vi "FGV_Analyse binary files.vi"(8 "error in (no error)":errorcluster, 9 "Funct data structure":bool, 11 "Get/Set info & refs":T1) -> (0 "Error out":errorcluster, 1 "Cam Binary Videos paths":path[](array[path]), 2 "Cam Binary Videos Refs":refnum<file>[](array[refnum]), 3 "Frame numbers & locations in each video file":T2[](array[typedef]))   [LabVIEW 2017]
uses:
  Typedefs/Number of frames and locations cluster.ctl
  Functional Imaging Viewer/Typedefs/Get-Set-Clear Control.ctl
  Globals/gl_Time series viewer globals.vi
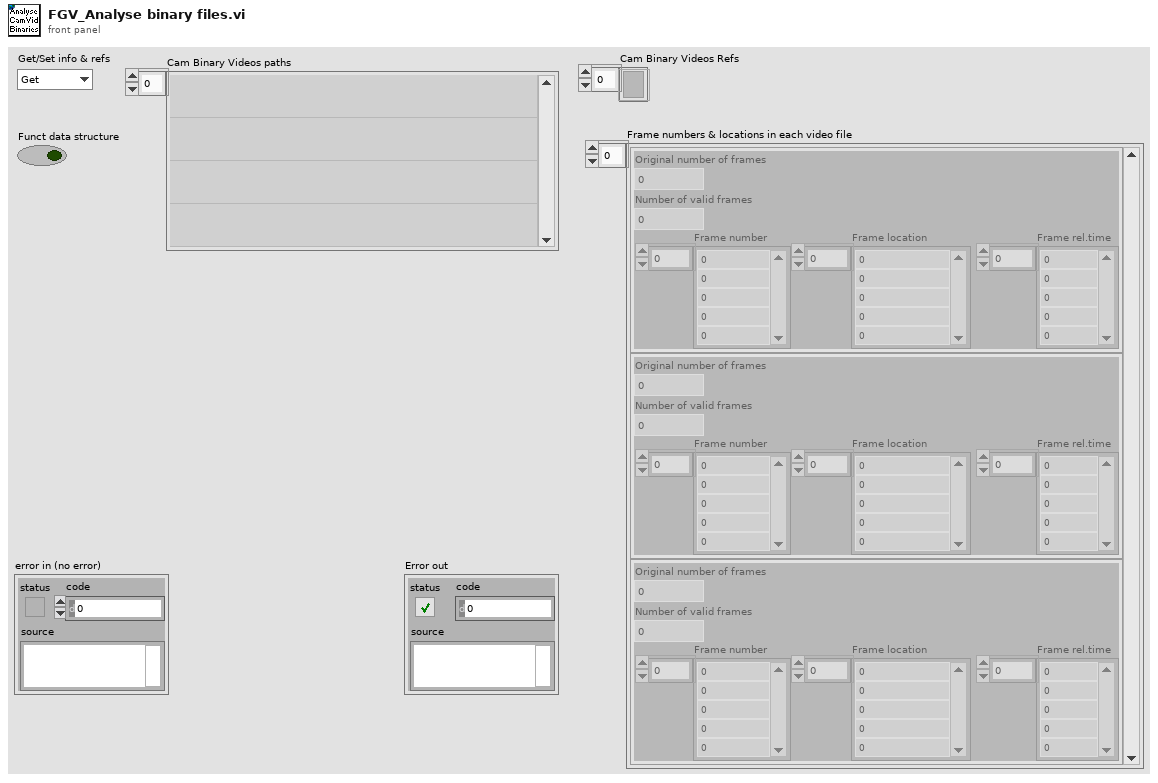
[diagram p1: front panel]
types:
  T1 = typedef "Get-Set-Clear Control.ctl" = enum16{"Get", "Set", "Clear"}
  T2 = typedef "Number of frames and locations cluster.ctl" = cluster{"Original number of frames":i32, "Number of valid frames":i32, "Frame number":i64[], "Frame location":i64[], "Frame rel.time":i64[]}
  T3 = typedef "Time series viewer refs.ctl" = cluster{"This VI":refnum<vi>, "Image control":refnum<vi>, "AVI Mode ind":refnum<vi>, "Play":refnum<vi>, "Stop":refnum<vi>, "Back":refnum<vi>, "Scrollbar":refnum<vi>, "Video length info":refnum<vi>, "Expected speed values":refnum<vi>, "Intensity":refnum<vi>, "Path":refnum<vi>, "Selection sliders":refnum<vi>, "Speed Graph ref":refnum<vi>, "Frame rate set (fps)":refnum<vi>, "Channel to load":refnum<vi>, "Number of rows to generate":refnum<vi>, "Colour":refnum<vi>}
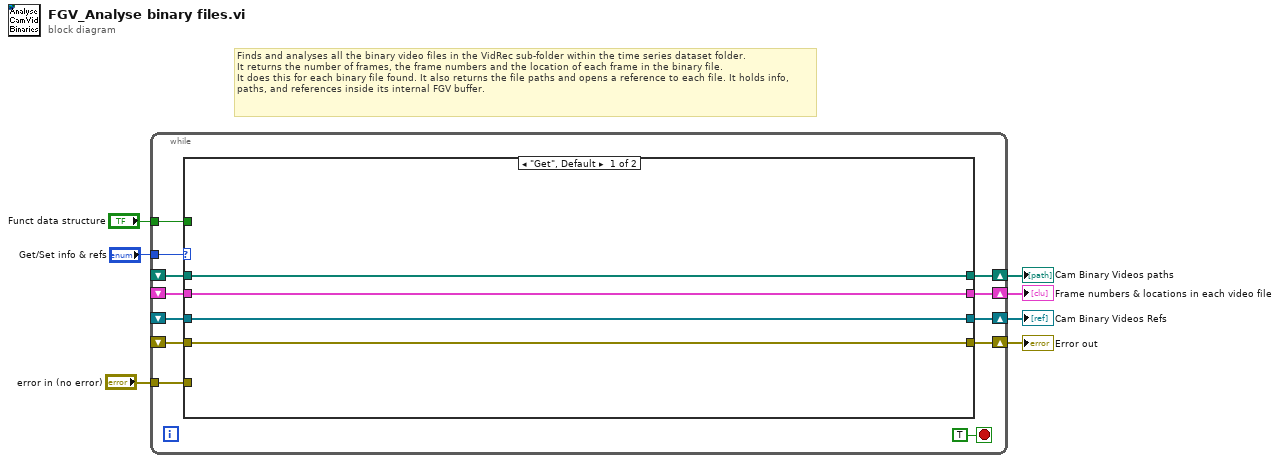
[diagram p0: block diagram]
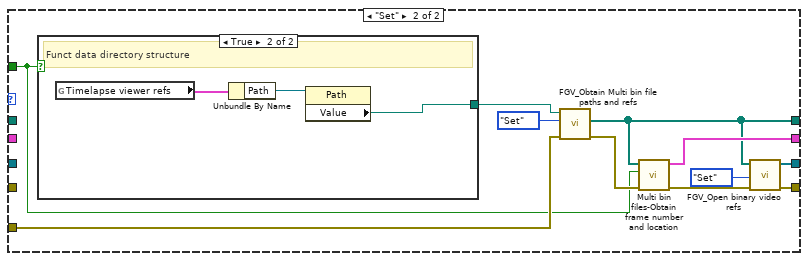
[diagram p2: hidden frame]
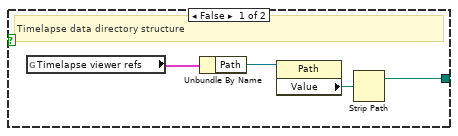
[diagram p3: hidden frame]
diagram:
  # "Finds and analyses all the binary video files in the VidRec sub-folder within the time series dataset folder.\nIt returns the number of frames, the frame numbers and the location of each frame in the binary file.\nIt does this for each binary file found. It also returns the file paths and opens a reference to each file. It holds info, paths, and references inside its internal FGV buffer."
  n1 = while {
    tunnel: "Get/Set info & refs" -> [w15]
    shift-right: [w18] -> w6
    shift-left: _ -> [w14]
    shift-right: [w19] -> w7
    shift-left: _ -> [w13]
    shift-right: [w17] -> w5
    shift-left: _ -> [w12]
    shift-right: [w11] -> w3
    shift-left: _ -> [w10]
    tunnel: "error in (no error)" -> [w9]
    tunnel: "Funct data structure" -> [w8]
    stop <- TRUE stop-if-true
    n2 = case shown="\"Get\", Default" w15 {
      tunnel: [w22 w34] -> w19
      tunnel: [w23 w32] -> w18
      tunnel: [w21 w31] -> w17
      tunnel: w14 -> [w23 _]
      tunnel: w13 -> [w22 _]
      tunnel: w12 -> [w21 _]
      tunnel: [w20 w26] -> w11
      tunnel: w10 -> [w20 _]
      tunnel: w9 -> [_ w25]
      tunnel: w8 -> [_ w24]
      frame "Get", Default {
      }
      frame "Set" {
        n3 = case shown="True" w24 {
          tunnel: [w35 w39] -> w29
          frame False {
            # "Timelapse data directory structure"
            n4 = global read "gl_Time series viewer globals.vi" "Timelapse viewer refs"() -> (w36:T3)
            n5 = Unbundle By Name(w36) -> ("Path"=w37:refnum<vi>)
            n6 = property class="Path"(reference=w37) -> ("Value"=w38:path)  [unwired: 1 in, 2 out]
            n7 = Strip Path(path=w38) -> (stripped path=w35:path)  [unwired: 1 out]
          }
          frame True {
            # "Funct data directory structure"
            n8 = global read "gl_Time series viewer globals.vi" "Timelapse viewer refs"() -> (w40:T3)
            n9 = Unbundle By Name(w40) -> ("Path"=w41:refnum<vi>)
            n10 = property class="Path"(reference=w41) -> ("Value"=w39:path)  [unwired: 1 in, 2 out]
          }
        }
        n11 = call "FGV_Obtain Multi bin file paths and refs.vi"("error in (no error)"=w25, "Function"=Get-Set-Clear_Control."Set", "Timelapse folder path"=w29) -> ("Error out"=w28:errorcluster, "Cam Binary Videos"=w26:path[])  [unwired: 7 in]
        n12 = call "Multi bin files-Obtain frame number and location.vi"("error in (no error)"=w28, "Funct data structure"=w24, "Cam Binary Videos paths"=w26) -> ("Error out"=w33:errorcluster, "Frame numbers & locations in each video file"=w32:T2[])  [unwired: 7 in]
        n13 = call "FGV_Open binary video refs.vi"("error in (no error)"=w33, "Function"=Get-Set-Clear_Control."Set", "Filtered Array in"=w26) -> ("error out"=w31:errorcluster, "Cam Binary Videos (ref)"=w34:refnum<file>[])  [unwired: 7 in]
      }
    }
  }
  "Cam Binary Videos Refs" <- w7
  "Frame numbers & locations in each video file" <- w6
  "Error out" <- w5
  "Cam Binary Videos paths" <- w3
